vi "Home one linear axis relative to limit DEMO.vi"() -> ()   [LabVIEW 2017]
panel:
  out "Response String ('/' codes)":string
  out "i":i32
  out "error out":errorcluster
  out "VISA resource out":refnum<visa-resource-name>
  in  "Set Home limit":bool caption="Set Home relative to this limit"
  in  "Axis (1..4)":u16(ring)=1 items=["X"=1, "Y"=2, "Z"=3, "Rotary"=4]
  in  "Absolute 0 position, counts":i32=2000 caption="Absolute 0 position from limit switch, counts"
  in  "VISA resource name":refnum<visa-resource-name>
  in  "stop":bool
  out "current position, counts":i32
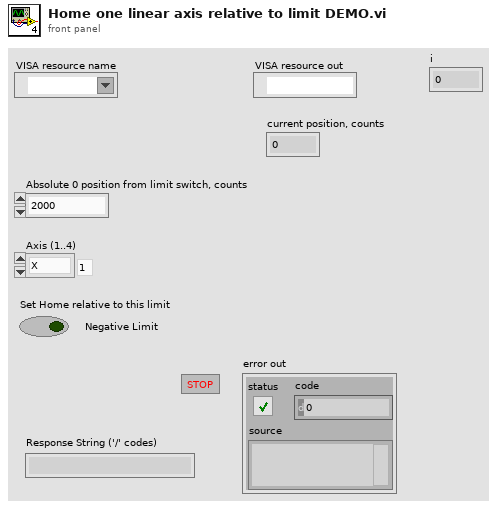
[diagram p1: front panel]
types:
  T1 = enum16{"Cmd-Response", "Write Only", "Read Only"}
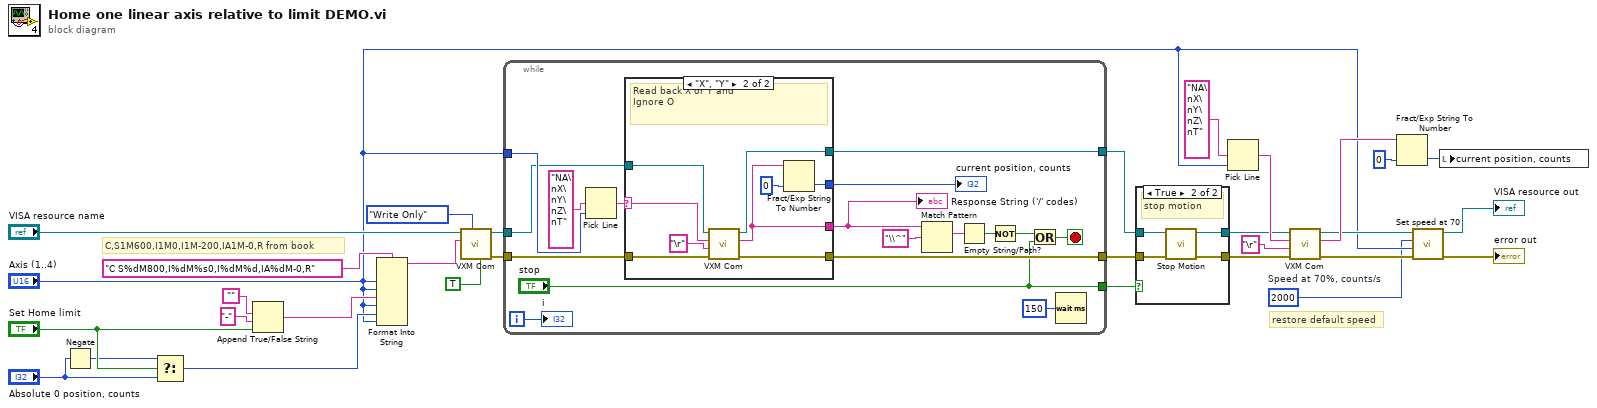
[diagram p0: block diagram]
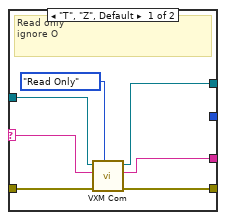
[diagram p3: hidden frame]
diagram:
  w7 = 2000  # Speed at 70%, counts/s
  # "restore default speed"
  # "C,S1M600,I1M0,I1M-200,IA1M-0,R from book"
  n1 = Negate(x="Absolute 0 position, counts") -> (-x=w20:i32)
  n2 = Select(t=w20, s="Set Home limit", f="Absolute 0 position, counts") -> (s? t:f=w23:i32)
  n3 = Append True/False String(1:"Set Home limit", 2:"-" ("false string"), 3:"") -> (0:w24:string)  [unwired: 1 in]
  n4 = Format Into String(format string="C S%dM800,I%dM%s0,I%dM%d,IA%dM-0,R" ("Write Buffer"), "Axis (1..4)", "Axis (1..4)", w24, "Axis (1..4)", w23, "Axis (1..4)") -> (resulting string=w19:string)  [unwired: 2 in, 1 out]
  n5 = call "VXM Com.vi"("Flush RS232"=TRUE, "Operation"=T1."Write Only", "Write Buffer ('/' codes)"=w19, "VISA resource name"="VISA resource name") -> ("error out"=w30:errorcluster, "VISA resource out"=w31:refnum<visa-resource-name>)  [unwired: 5 in, 1 out]
  n6 = while {
    tunnel: "Axis (1..4)" -> [w47]
    tunnel: w31 -> [w43]
    tunnel: w30 -> [w42]
    tunnel: [w37] -> w6
    tunnel: [w36] -> w4
    tunnel: ["stop"] -> w2
    i -> [w35]
    stop <- w38 stop-if-true
    n7 = Pick Line(multi-line string="NA\nX\nY\nZ\nT", line index=w47) -> (output string=w32:string)  [unwired: 1 in]
    n8 = case shown="\"X\", \"Y\"" w32 {
      selector: w32 -> [w50 w56]
      tunnel: [_ w62] -> w45
      tunnel: [w55 w61] -> w44
      tunnel: w43 -> [w54 w60]
      tunnel: w42 -> [w53 w59]
      tunnel: [w52 w58] -> w37
      tunnel: [w51 w57] -> w36
      frame "T", "Z", Default {
        # "Read only ^\nignore O"
        n9 = call "VXM Com.vi"("Operation"=T1."Read Only", "error in (no error)"=w53, "Write Buffer ('/' codes)"=w50, "VISA resource name"=w54) -> ("error out"=w52:errorcluster, "Response String ('/' codes)"=w55:string, "VISA resource out"=w51:refnum<visa-resource-name>)  [unwired: 5 in]
      }
      frame "X", "Y" {
        # "Read back X or Y and ^\nIgnore O"
        n10 = call "VXM Com.vi"("error in (no error)"=w59, "Termination String ('/' codes)"="\r", "Write Buffer ('/' codes)"=w56, "VISA resource name"=w60) -> ("error out"=w58:errorcluster, "Response String ('/' codes)"=w61:string, "VISA resource out"=w57:refnum<visa-resource-name>)  [unwired: 5 in]
        n11 = Fract/Exp String To Number(string=w61, default (0 dbl)=0 ("default (0 DBL)")) -> (number=w62:i32)  [unwired: 2 in, 1 out]
      }
    }
    "current position, counts" <- w45
    "Response String ('/' codes)" <- w44
    n12 = Match Pattern(string=w44, regular expression="\\^") -> (match substring=w41:string)  [unwired: 1 in, 3 out]
    n13 = Empty String/Path?(string/path=w41) -> (empty?=w40:bool)
    n14 = Not(x=w40) -> (.not. x?=w39:bool)
    n15 = Or(x=w39, y="stop") -> (x .or. y?=w38:bool)
    n16 = Wait (ms)(milliseconds to wait=u32 150) -> ()  [unwired: 1 out]
    "i" <- w35
  }
  n17 = case shown="True" w2 {
    tunnel: w6 -> [w66 w70]
    tunnel: [w66 w69] -> w5
    tunnel: w4 -> [w65 w68]
    tunnel: [w65 w67] -> w3
    frame False {
    }
    frame True {
      # "stop motion"
      n18 = call "Stop Motion.vi"("error in (no error)"=w70, "VISA resource name"=w68) -> ("error out"=w69:errorcluster, "VISA resource out"=w67:refnum<visa-resource-name>)  [unwired: 8 in]
    }
  }
  n19 = Pick Line(multi-line string="NA\nX\nY\nZ\nT", line index="Axis (1..4)") -> (output string=w14:string)  [unwired: 1 in]
  n20 = call "VXM Com.vi"("error in (no error)"=w5, "Termination String ('/' codes)"="\r", "Write Buffer ('/' codes)"=w14, "VISA resource name"=w3) -> ("error out"=w11:errorcluster, "Response String ('/' codes)"=w16:string, "VISA resource out"=w10:refnum<visa-resource-name>)  [unwired: 5 in]
  n21 = Fract/Exp String To Number(string=w16, default (0 dbl)=0 ("default (0 DBL)")) -> (number=w13:i32)  [unwired: 2 in, 1 out]
  n22 = call "Set speed at 70.vi"("error in (no error)"=w11, "Axis (1..4)"="Axis (1..4)", "Speed at 70%, counts/s"=w7, "VISA resource name"=w10) -> ("error out"=→"error out":errorcluster, "VISA resource out"=→"VISA resource out":refnum<visa-resource-name>)  [unwired: 6 in]
  n23 = local write "current position, counts"(w13) -> ()
